vi "PH_Class.Register Event.vi"(0 "i ref in":refnum<vi>, 5 "error in (no error)":errorcluster) -> (14 "i ref out":refnum<vi>, 17 "Event Registration Refnum":refnum<event-registration>, 19 "error out":errorcluster)   [LabVIEW 2014, in "PH_Class.lvlib"]
uses:
  PH_Class.lvlib
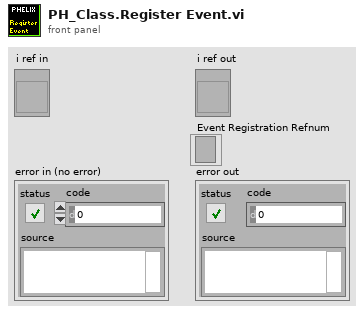
[diagram p1: front panel]
types:
  T1 = typedef "PH_Class.lvlib/PH_Class.i attribute.ctl" = cluster{"Event":refnum<user-event>, "Event registered":refnum<k4>, "GUI Refs stored":refnum<k4>}
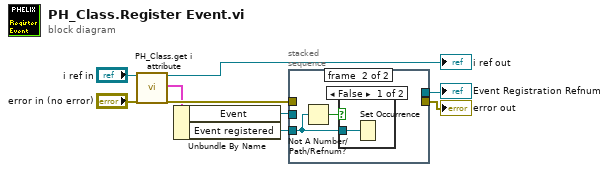
[diagram p0: block diagram]
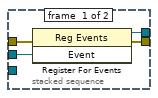
[diagram p2: hidden frame]
diagram:
  n1 = call "PH_Class.get i attribute.vi"("i ref in"="i ref in", "error in (no error)"="error in (no error)") -> ("i ref out"=→"i ref out":refnum<vi>, "i attribute"=w3:T1, "error out"=w4:errorcluster)  [unwired: 15 in]
  n2 = Unbundle By Name(w3) -> ("Event"=w9:refnum<user-event>, "Event registered"=w6:refnum<k4>)
  n3 = stacked-sequence {
    tunnel: w9 -> [w13 _]
    tunnel: w4 -> [w12 _]
    tunnel: [w11 _] -> w7
    tunnel: [w10 _] -> w5
    tunnel: w6 -> [_ w15]
    frame #0 {
      n4 = register-events(error in=w12, w13) -> (reference out=w10:refnum<event-registration>, error out=w11:errorcluster)  [unwired: 1 in]
    }
    frame #1 {
      n5 = Not A Number/Path/Refnum?(number/path/refnum=w15) -> (NaN/Path/Refnum?=w14:bool)
      n6 = case shown="False" w14 {
        tunnel: w15 -> [w16 _]
        frame False {
          n7 = Set Occurrence(w16) -> ()
        }
        frame True {
        }
      }
    }
  }
  "error out" <- w7
  "Event Registration Refnum" <- w5
